vi "Module example event handler inside.vi"() -> ()   [LabVIEW 2021, in "MessengerLib.lvlib"]
uses:
  MessengerLib.lvlib
  Data types/Mailbox address.ctl
  Data types/Module name.ctl
  Data types/MSG to TOP.ctl
panel:
  in  "error in":errorcluster
  in  "timeout":i32=-1
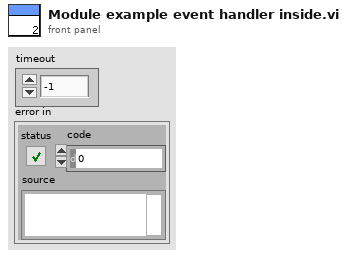
[diagram p1: front panel]
types:
  T1 = enum16{"Start", "Wait for message", "Wait for event", "Stop", "Close"}
  T2 = typedef "MessengerLib.lvlib/Mailbox address.ctl" = refnum<queue>
  T3 = typedef "MessengerLib.lvlib/MSG to TOP.ctl" = cluster{"Module":T4, "Response":string, "Data":variant, "Time":timestamp}
  T4 = typedef "MessengerLib.lvlib/Module name.ctl" = enum16{"Emty", "Magnet", "VTI", "Excitation", "Servo", "Acquisition", "Rotator", "Digitizer", "SMU2450", "Carousel", "Multimeter", "Tmp monitor", "Power monitor"}
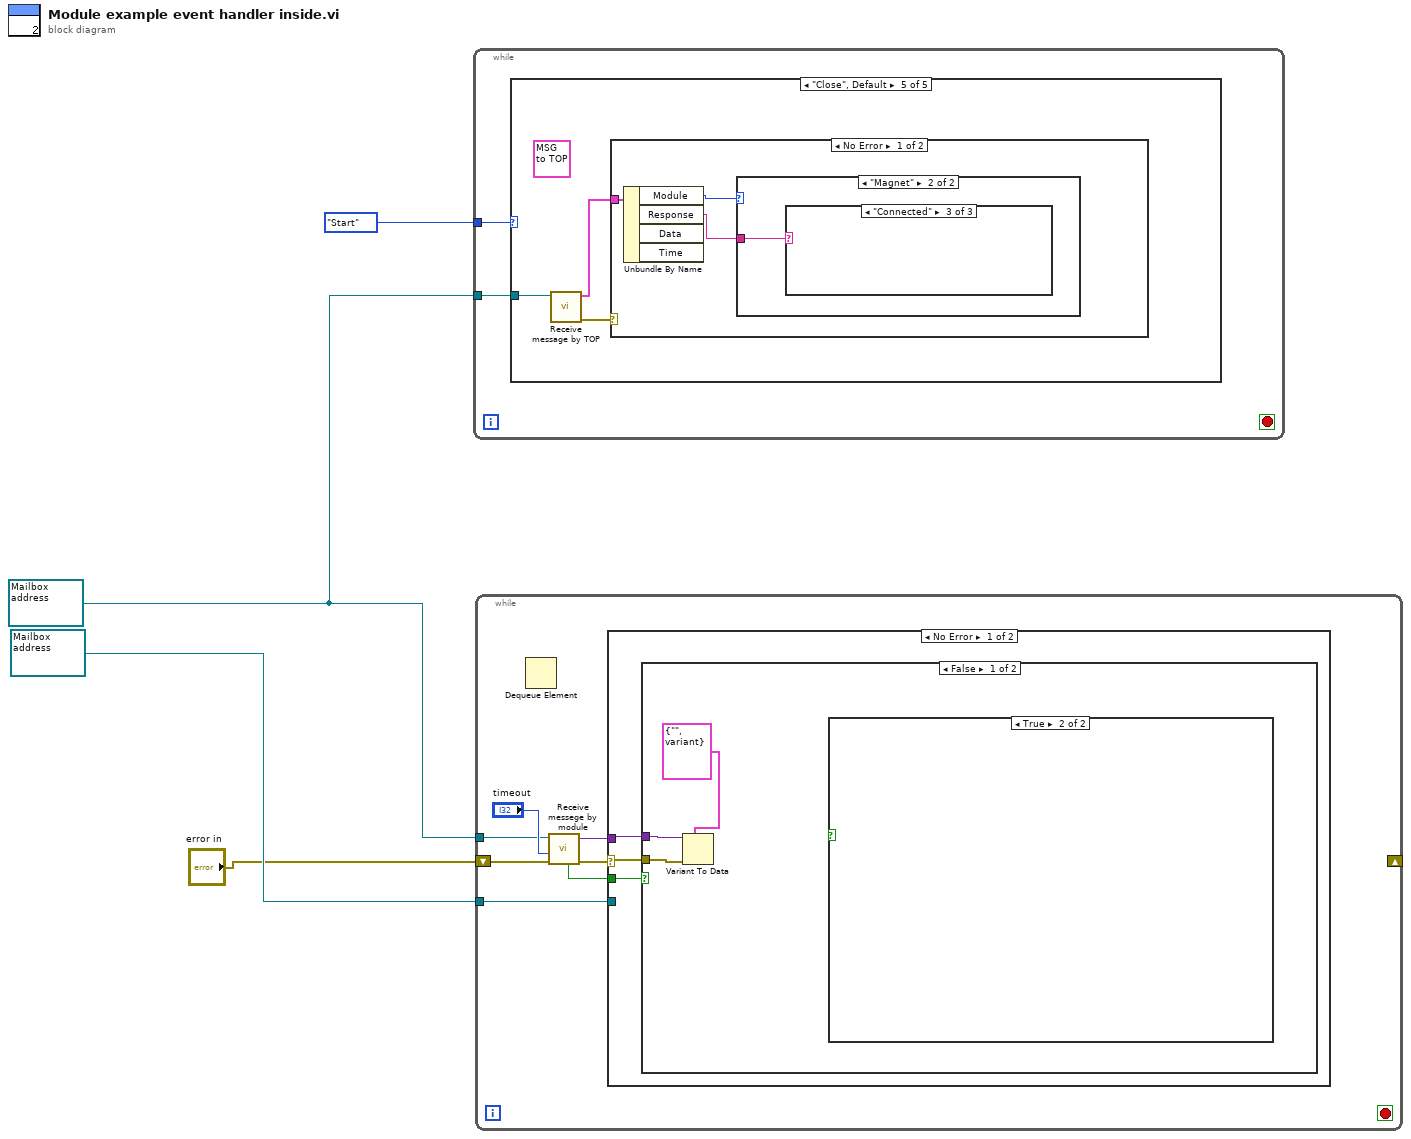
[diagram p0: block diagram]
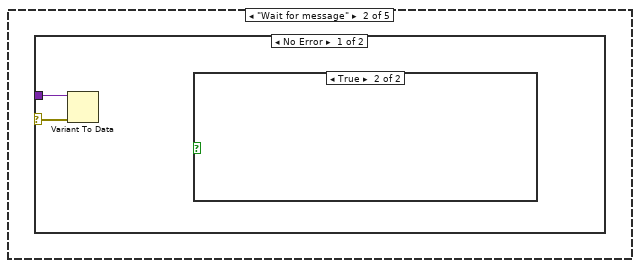
[diagram p3: hidden frame]
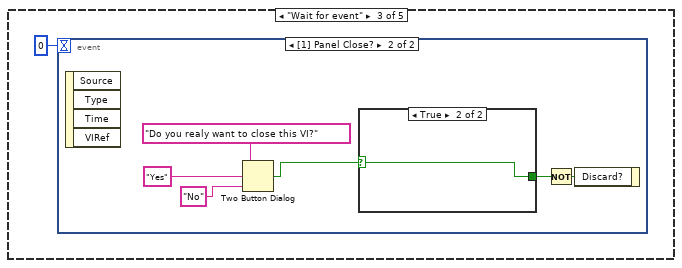
[diagram p6: hidden frame]
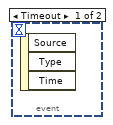
[diagram p7: hidden frame]
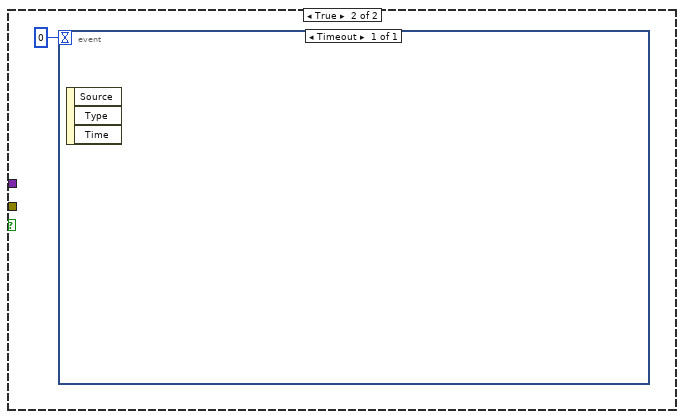
[diagram p15: hidden frame]
diagram:
  w1 = T2 refnum ("Module mailbox")
  n1 = while {
    tunnel: T1."Start" -> [w6]
    tunnel: w1 -> [w5]
    stop <- _ stop-if-true
    n2 = case shown="\"Close\", Default" w6 {
      tunnel: w5 -> [_ _ _ _ w20]
      frame "Start" {
      }
      frame "Wait for message" {
        n3 = case shown="No Error" {
          selector: _ -> [w7 _]
          tunnel: _ -> [w8 _]
          frame No Error {
            n4 = Variant To Data(error in=w7, Variant=w8) -> ()  [unwired: 1 in, 2 out]
            n5 = case shown="True" {
              selector: _ -> [_ _]
              frame False {
              }
              frame True {
              }
            }
          }
          frame Error {
          }
        }
      }
      frame "Wait for event" {
        n6 = event shown="[1] Panel Close?" {
          selector: _ -> [_ _]
          dyn-events: _ -> [_ _]
          timeout: 0 -> [_ _]
          event Timeout {
            n7 = event-data() -> ()  [unwired: 1 in, 3 out]
          }
          event Panel Close? {
            n8 = event-data() -> ()  [unwired: 1 in, 4 out]
            n9 = Two Button Dialog(message="Do you realy want to close this VI?", 1:"No" ("T button name (\"OK\")"), 2:"Yes" ("T button name (\"OK\")")) -> (T button?=w11:bool)
            n10 = case shown="True" w11 {
              selector: w11 -> [w16 w17]
              tunnel: [w16 w17] -> w10
              frame False {
              }
              frame True {
              }
            }
            n11 = Not(x=w10) -> (.not. x?=w12:bool)
            n12 = event-data("Discard?"=w12) -> ()  [unwired: 1 in, 1 out]
          }
        }
      }
      frame "Stop" {
      }
      frame "Close", Default {
        (unwired) T3 {"Module"=enum."Emty", "Response"="", "Data"=variant, "Time"=timestamp(0 s since 1904-01-01)} ("MSG packet")
        n13 = call "Receive message by TOP.vi"("Mailbox in"=w20) -> ("error out"=w18:errorcluster, "MSG packet"=w19:T3)  [unwired: 7 in, 2 out]
        n14 = case shown="No Error" w18 {
          tunnel: w19 -> [w23 _]
          frame No Error {
            n15 = Unbundle By Name(w23) -> ("Module"=w22:T4, "Response"=w21:string)  [unwired: 2 out]
            n16 = case shown="\"Magnet\"" w22 {
              tunnel: w21 -> [_ w24]
              frame "Emty", Default {
              }
              frame "Magnet" {
                n17 = case shown="\"Connected\"" w24 {
                  frame "Ignore", Default {
                  }
                  frame "Error" {
                  }
                  frame "Connected" {
                  }
                }
              }
            }
          }
          frame Error {
          }
        }
      }
    }
  }
  n18 = while {
    tunnel: T2 refnum ("Mailbox address in") -> [w31]
    tunnel: w1 -> [w29]
    shift-right: _ -> [_]
    shift-left: "error in" -> [w27]
    stop <- _ stop-if-true
    n19 = Dequeue Element() -> ()  [unwired: 3 in, 4 out]
    n20 = call "Receive messege by module.vi"("error in (no error)"=w27, "timeout in ms (-1)"="timeout", "Module mailbox"=w29) -> ("error out"=w26:errorcluster, "Data"=w28:variant, "timed out?"=w25:bool)  [unwired: 4 in, 2 out]
    n21 = case shown="No Error" w26 {
      selector: w26 -> [w32 _]
      tunnel: w31 -> [_ _]
      tunnel: w28 -> [w33 _]
      tunnel: w25 -> [w34 _]
      frame No Error {
        n22 = case shown="False" w34 {
          tunnel: w33 -> [w37 _]
          tunnel: w32 -> [w36 _]
          frame False {
            n23 = Variant To Data(error in=w36, type=cluster{enum16{""}, variant} {enum."", variant}, Variant=w37) -> ()  [unwired: 2 out]
            n24 = case shown="True" {
              selector: _ -> [_ _]
              frame False {
              }
              frame True {
              }
            }
          }
          frame True {
            n25 = event shown="[0] Timeout" {
              selector: _ -> [_]
              dyn-events: _ -> [_]
              timeout: 0 -> [_]
              event Timeout {
                n26 = event-data() -> ()  [unwired: 1 in, 3 out]
              }
            }
          }
        }
      }
      frame Error {
      }
    }
  }
